vi "Json_Data_Path_Argentina.vi"(2 "Json File Path":path, 5 "ERD Data In":cluster{"ERD Number":u16, "Data":string}[](array[cluster]) {"ERD Number" format="%.0x"}, 11 "error in":errorcluster) -> (6 "ERD Data Out":cluster{"ERD Number":u16, "Data":string}[](array[cluster]) {"ERD Number" format="%.0x"}, 15 "error out":errorcluster)   [LabVIEW 2021]
uses:
  <vilib>/JDP Science/JSONtext/String Subset.vi
  <vilib>/JDP Science/JSONtext/support/Strip Quotes and Unescape.vi
  <vilib>/JDP Science/JSONtext/support/Unescape JSON string.vi
  <vilib>/JDP Science/JSONtext/Parsing/Parse Full Path or Item Name.vi
  <vilib>/JDP Science/JSONtext/Offset/Find Item Locations by Path.vi
  <vilib>/JDP Science/JSONtext/JSONtext.lvlib
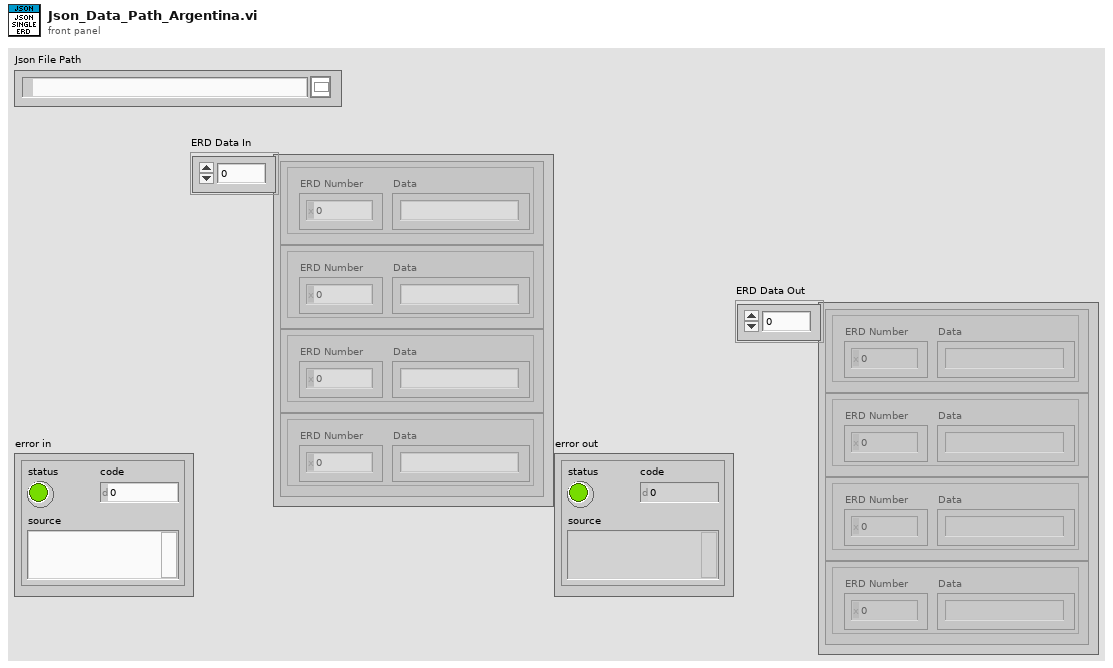
[diagram p1: front panel]
types:
  T1 = enum16{"open", "replace", "create", "open or create", "replace or create", "replace or create with confirmation"}
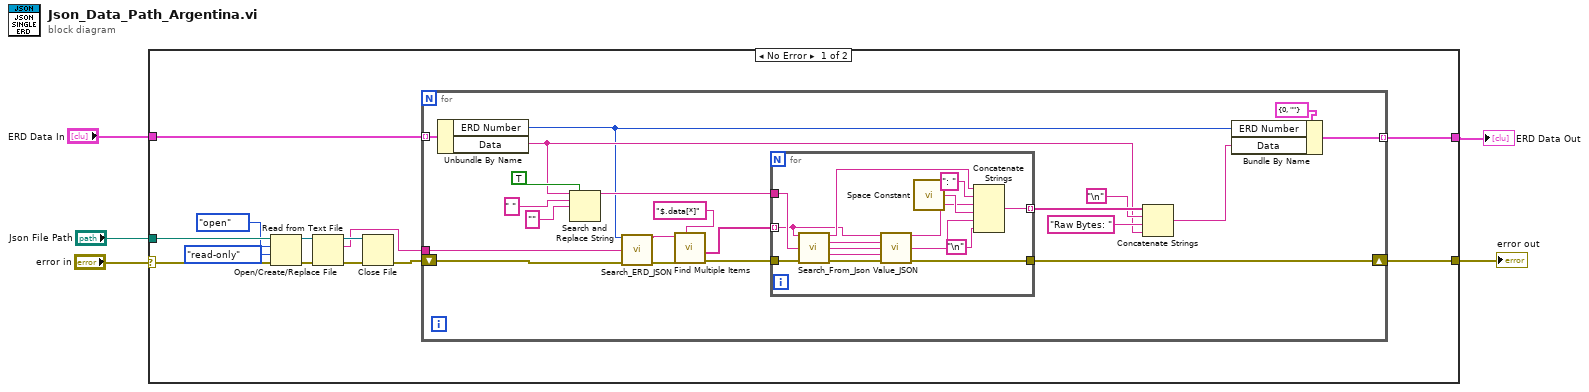
[diagram p0: block diagram]
diagram:
  n1 = case shown="No Error" "error in" {
    selector: "error in" -> [w13 w55]
    tunnel: [w10 w55] -> w4
    tunnel: "Json File Path" -> [w14 _]
    tunnel: [w6 _] -> w1
    tunnel: "ERD Data In" -> [w7 _]
    frame No Error {
      n2 = Open/Create/Replace File(file path (use dialog)=w14, error in=w13, operation (0:open)=T1."open", access (0:read/write)=enum16{"read/write", "read-only", "write-only"}."read-only") -> (refnum out=w16:refnum<file>, error out=w18:errorcluster)  [unwired: 2 in, 1 out]
      n3 = Read from Text File(file (use dialog)=w16, error in=w18) -> (refnum out=w15:refnum<file>, text=w11:string, error out=w17:errorcluster)  [unwired: 2 in, 1 out]
      n4 = Close File(refnum=w15, error in=w17) -> (error out=w12:errorcluster)  [unwired: 1 out]
      n5 = for {
        tunnel: w11 -> [w30]
        shift-right: [w28] -> w10
        shift-left: w12 -> [w31]
        tunnel: w7 -> [w23] mode=indexing
        tunnel: [w21] -> w6 mode=indexing
        n6 = Unbundle By Name(w23) -> ("ERD Number"=w22:u16, "Data"=w24:string)
        n7 = Search and Replace String(replace all?=TRUE ("replace all? (F)"), input string=w24, search string=" ", replace string="" ("replace string (\"\")")) -> (result string=w29:string)  [unwired: 4 in, 3 out]
        n8 = call "Search_ERD_JSON.vi"("ERD Number"=w22, "JSON Text"=w30, "error in"=w31) -> ("ERD"=w33:string, "error out"=w34:errorcluster)  [unwired: 11 in]
        n9 = call <vilib>:"Find Multiple Items.vi"("$Path or Item Name"="$.data[*]", "error in (no error)"=w34, "JSON"=w33) -> ("error out"=w32:errorcluster, "<JSON>"=w38:string[])  [unwired: 5 in, 2 out]
        n10 = for {
          tunnel: w38 -> [w49] mode=indexing
          tunnel: w29 -> [w51]
          tunnel: [w52] -> w27 mode=indexing
          tunnel: [w42] -> w28
          tunnel: w32 -> [w41]
          n11 = call "Search_From_Json.vi"("Data JSON"=w49, "ERD"=w51, "error in"=w41) -> ("Name"=w50:string, "Type"=w48:string, "Size data"=w47:string, "Hexa"=w46:string, "error IO"=w45:errorcluster)  [unwired: 8 in]
          n12 = call "Value_JSON.vi"("Data JSON"=w49, "Type"=w48, "Size data"=w47, "Hexa"=w46, "error in"=w45) -> ("Value_string"=w44:string, "Hexa value"=w43:string, "error IO"=w42:errorcluster)  [unwired: 8 in]
          n13 = call <vilib>:"Space Constant.vi"() -> ("String"=w53:string)
          n14 = Concatenate Strings(w50, ": " ("string"), w44, w53, w43, "\n") -> (w52:string)
        }
        n15 = Concatenate Strings(w27, "\n", "Raw Bytes: " ("string"), w24) -> (w19:string)
        n16 = Bundle By Name(cluster=cluster{"ERD Number":u16, "Data":string} {"ERD Number"=0, "Data"=""} ("ERD Cluster"), "ERD Number"=w22, "Data"=w19) -> (w21:cluster{"ERD Number":u16, "Data":string})
      }
    }
    frame Error {
    }
  }
  "error out" <- w4
  "ERD Data Out" <- w1
